vi "CustomView.vi"(8 "error in":errorcluster, 10 "View Name":string, 11 "SequenceRepo in":refnum<class "SequenceRepo.lvclass">) -> (0 "error out":errorcluster, 3 "SequenceRepo out":refnum<class "SequenceRepo.lvclass">)   [LabVIEW 2015, in "SequenceRepo.lvclass"]
doc: "Copyright 2017 National Instruments Corporation\n\nLicensed under the Apache License, Version 2.0 (the \"License\"); you may not use this file except in compliance with the License. You may obtain a copy of the License at http://www.apache.org/licenses/LICENSE-2.0\nUnless required by applicable law or agreed to in writing, software distributed under the License is distributed on an \"AS IS\" BASIS, WITHOUT WARRANTIES OR CONDITIONS OF ANY KIND, either express or implied. See the License for the specific language governing permissions and limitations under the License."
uses:
  SequenceRepo.lvclass
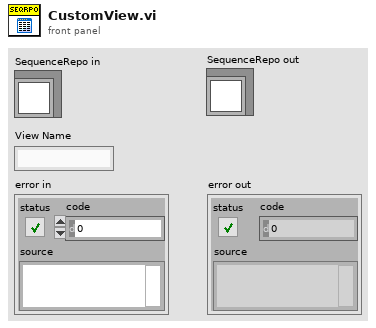
[diagram p1: front panel]
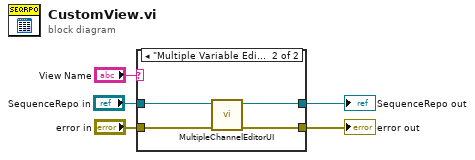
[diagram p0: block diagram]
diagram:
  n1 = case shown="\"Multiple Variable Editor\"" "View Name" {
    tunnel: "SequenceRepo in" -> [w7 w11]
    tunnel: "error in" -> [w6 w10]
    tunnel: [w6 w9] -> w3
    tunnel: [w7 w8] -> w2
    frame "False", Default {
    }
    frame "Multiple Variable Editor" {
      n2 = call "MultipleChannelEditorUI.vi"("error in"=w10, "SequenceRepo in"=w11) -> ("error out"=w9:errorcluster, "SequenceRepo out"=w8:refnum<class "SequenceRepo.lvclass">)  [unwired: 8 in]
    }
  }
  "SequenceRepo out" <- w2
  "error out" <- w3
